vi "ICCD Noise Data Viewer.vi"() -> ()   [LabVIEW 2021, in "AlliGator Camera Noise Influence on Lifetime.lvlib"]
uses:
  AlliGator Camera Noise Influence on Lifetime.lvlib
  Decay Fit Parameter Map/AlliGator Power Law Fit Results.ctl
  Power Law Parameters.ctl
  ICCD Parameter Set.ctl
  Utilities/Utilities.lvlib
  Graphs/XY Graph/XY Graph Add-Ons.lvlib
  <vilib>/Utility/miscctls.llb/LVPoint32TypeDef.ctl
  Graphs/XY Graph/XY Graph Event.ctl
panel:
  out "LabVIEW PL+B":T1={"Power Law Parameters"={"amplitude"=1354.9125948149328, "power"=-1.4827495284911292, "offset"=0.013950226554821962}, "R^2"=0.9896721333021318, "Chi^2"=0.00026681950170242603}
  in  "Abscissa":enum32{"I-", "<I>"}(radio)=enum."<I>"
  out "error out":T3
  out "Data":T1={"Power Law Parameters"={"amplitude"=20.050788088429826, "power"=-0.808279791250982, "offset"=0.0}, "R^2"=0.9320325995197519, "Chi^2"=0.0015050842644887775}
  out "LabVIEW PL":T1={"Power Law Parameters"={"amplitude"=1354.9125919047456, "power"=-1.4228141762361315, "offset"=0.0}, "R^2"=0.6411917195333446, "Chi^2"=0.007945525253030357}
  out "File Name":string="Bin1_MCP560_Power300_Exp100_alligator_sliced"
  out "XY Graph":cluster{"X Array":dbl[], "Y Array":dbl[]}[](graph)=[{"X Array"=[589.8712230215828, 1449.84, 2492.5444234404536, 3505.6867469879517, 4503.983673469388, 5488.8125, 6478.855626326964, 7416.982608695652, 8415.288], "Y Array"=[0.12017889524722658, 0.04584267100112674, 0.02646477188778284, 0.021275407414964982, 0.018663783988422344, 0.018541333295241307, 0.013827404460717034, 0.016008850611953694, 0.01898370316876584]}, {"X Array"=[589.8712230215828, 1449.84, 2492.5444234404536, 3505.6867469879517, 4503.983673469388, 5488.8125, 6478.855626326964, 7416.982608695652, 8415.288], "Y Array"=[0.1155004849822888, 0.05583411708587998, 0.03603237727021303, 0.027350309068035653, 0.022335836275987765, 0.019036444971124028, 0.01664844199637044, 0.01492464998854605, 0.013476486701475781]}, {"X Array"=[589.8712230215828, 1449.84, 2492.5444234404536, 3505.6867469879517, 4503.983673469388, 5488.8125, 6478.855626326964, 7416.982608695652, 8415.288], "Y Array"=[0.15475284512882467, 0.04304673899987971, 0.019912216190079178, 0.012256256772752168, 0.008580684756946514, 0.0064763215930010035, 0.005115139257444052, 0.0042198505196813525, 0.0035258796664633094]}, {"X Array"=[589.8712230215828, 1449.84, 2492.5444234404536, 3505.6867469879517, 4503.983673469388, 5488.8125, 6478.855626326964, 7416.982608695652, 8415.288], "Y Array"=[0.11952795988993804, 0.041777164889661475, 0.026410874061133384, 0.021464735869369332, 0.019132762657076766, 0.017815688947243814, 0.016973058263863076, 0.01642385025852421, 0.016001469474992334]}]
  in  "MCP Voltage (V)":i32(ring)=2 items=["460", "510", "560", "610"]
  in  "Laser Power (mW)":i32(ring)=2 items=["100", "200", "300", "400", "500", "600"]
  in  "Exposure (ms)":i32(ring) items=["100", "200", "300", "400", "500"]
  in  "Binning":i32(ring) items=["1", "2", "4"]
  in  "Analysis Data Folder":path=path "D:/UCLA Thinkpad Google Drive/Work/Manuscripts/2025/OL 2025 (ICCD Lifetime CV)/Material/Intensity sliced"
  in  "Parameter File":path=path "D:/UCLA Thinkpad Google Drive/Work/Manuscripts/2025/OL 2025 (ICCD Lifetime CV)/Material/LUT.xlsx"
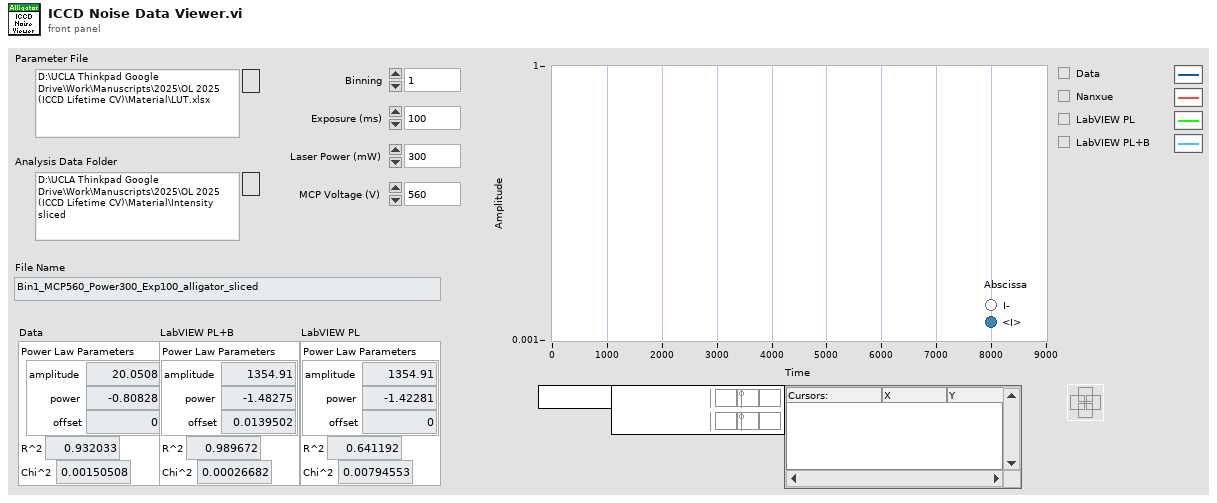
[diagram p1: front panel]
types:
  T1 = typedef "AlliGator Camera Noise Influence on Lifetime.lvlib/AlliGator Power Law Fit Results.ctl" = cluster{"Power Law Parameters":T2, "R^2":dbl, "Chi^2":dbl}
  T2 = typedef "AlliGator Camera Noise Influence on Lifetime.lvlib/Power Law Parameters.ctl" = cluster{"amplitude":dbl, "power":dbl, "offset":dbl}
  T3 = cluster{"status":bool, "Error Code":i32, "source":string}
  T4 = typedef "XY Graph Add-Ons.lvlib/XY Graph Event.ctl" = cluster{"Item Tag":string, "XY Graph Refnum":refnum<vi>, "Coords":T5, "Item Path":string}
  T5 = typedef "LVPoint32TypeDef.ctl" = cluster{"Horizontal":i32, "Vertical":i32}
  T6 = typedef "AlliGator Camera Noise Influence on Lifetime.lvlib/ICCD Parameter Set.ctl" = cluster{"Binning":refnum<vi>, "Exposure (ms)":refnum<vi>, "Laser Power (mW)":refnum<vi>, "MCP Voltage (V)":refnum<vi>}
  T7 = typedef "XY Graph Add-Ons.lvlib/XY Graph Plot Data.ctl" = cluster{"X Array":dbl[], "Y Array":dbl[]}
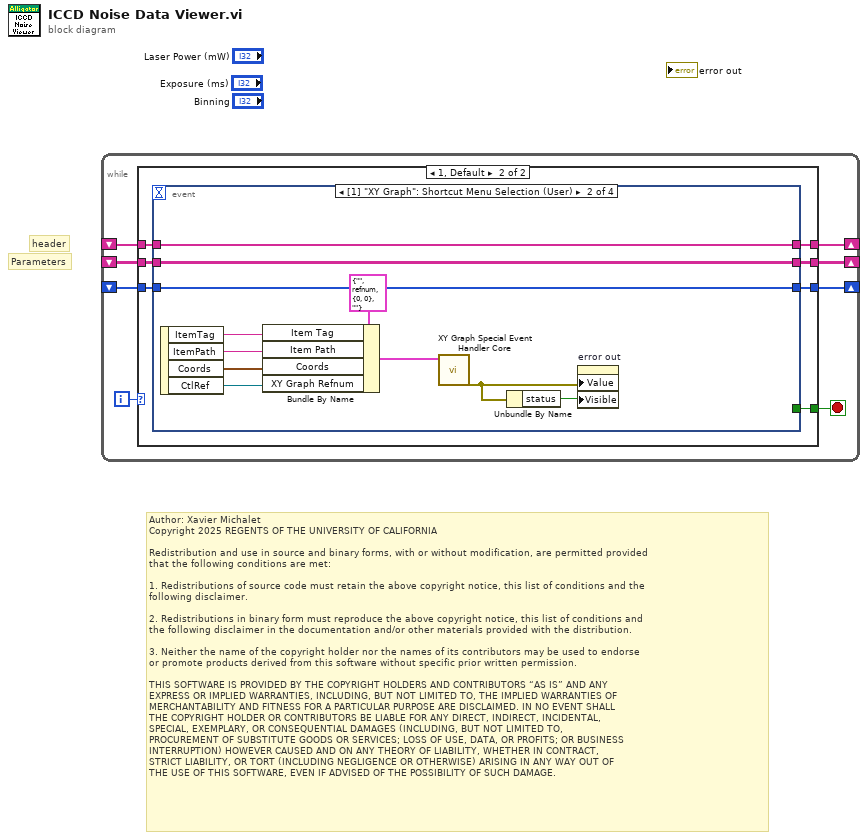
[diagram p0: block diagram]
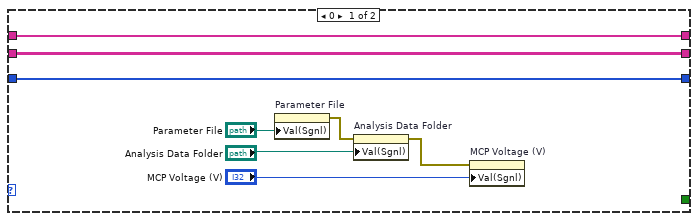
[diagram p2: hidden frame]
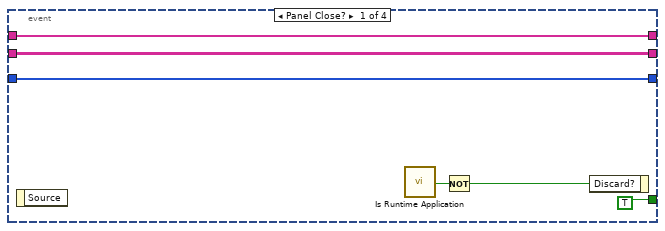
[diagram p3: hidden frame]
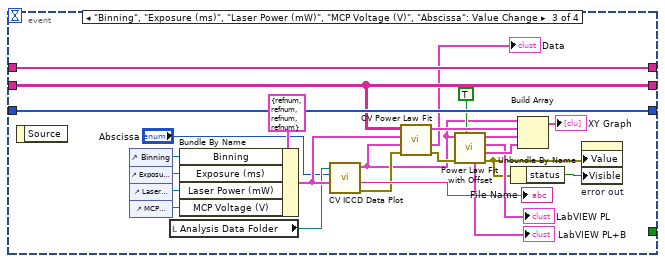
[diagram p4: hidden frame]
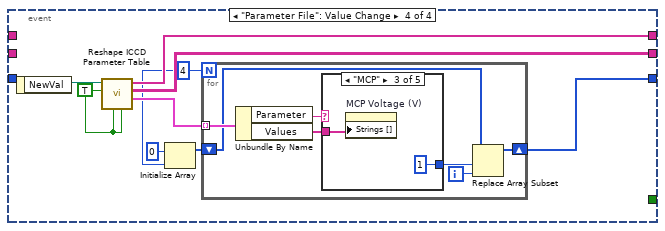
[diagram p5: hidden frame]
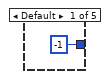
[diagram p6: hidden frame]
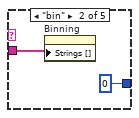
[diagram p7: hidden frame]
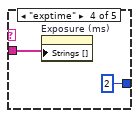
[diagram p8: hidden frame]
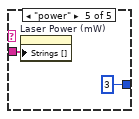
[diagram p9: hidden frame]
diagram:
  # "Author: Xavier Michalet\nCopyright 2025 REGENTS OF THE UNIVERSITY OF CALIFORNIA\n\nRedistribution and use in source and binary forms, with or without modification, are permitted provided\nthat the following conditions are met:\n\n1. Redistributions of source code must retain the above copyright notice, this list of conditions and the\nfollowing disclaimer.\n\n2. Redistributions in binary form must reproduce the above copyright notice, this list of conditions and\nthe following disclaimer in the documentation and/or other materials provided with the distribution.\n\n3. Neither the name of the copyright holder nor the names of its contributors may be used to endorse \nor promote products derived from this software without specific prior written permission.\n\nTHIS SOFTWARE IS PROVIDED BY THE COPYRIGHT HOLDERS AND CONTRIBUTORS “AS IS” AND ANY \nEXPRESS OR IMPLIED WARRANTIES, INCLUDING, BUT NOT LIMITED TO, THE IMPLIED WARRANTIES OF\nMERCHANTABILITY AND FITNESS FOR A PARTICULAR PURPOSE ARE DISCLAIMED. IN NO EVENT SHALL\nTHE COPYRIGHT HOLDER OR CONTRIBUTORS BE LIABLE FOR ANY DIRECT, INDIRECT, INCIDENTAL, \nSPECIAL, EXEMPLARY, OR CONSEQUENTIAL DAMAGES (INCLUDING, BUT NOT LIMITED TO, \nPROCUREMENT OF SUBSTITUTE GOODS OR SERVICES; LOSS OF USE, DATA, OR PROFITS; OR BUSINESS\nINTERRUPTION) HOWEVER CAUSED AND ON ANY THEORY OF LIABILITY, WHETHER IN CONTRACT, \nSTRICT LIABILITY, OR TORT (INCLUDING NEGLIGENCE OR OTHERWISE) ARISING IN ANY WAY OUT OF\nTHE USE OF THIS SOFTWARE, EVEN IF ADVISED OF THE POSSIBILITY OF SUCH DAMAGE."
  # "Parameters"
  # "header"
  n1 = while {
    shift-right: [w7] -> _
    shift-left: _ -> [w3]
    shift-right: [w6] -> _
    shift-left: _ -> [w4]
    shift-right: [w5] -> _
    shift-left: _ -> [w2]
    i -> [w1]
    stop <- w8 stop-if-true
    n2 = case shown="1, Default" w1 {
      tunnel: [_ w23] -> w8
      tunnel: [w10 w22] -> w7
      tunnel: [w11 w21] -> w6
      tunnel: [w9 w20] -> w5
      tunnel: w4 -> [w11 w19]
      tunnel: w3 -> [w10 w18]
      tunnel: w2 -> [w9 w17]
      frame 0 {
        n3 = property on="Parameter File" class="Path"("Val(Sgnl)"="Parameter File") -> (error out=w15:errorcluster)  [unwired: 2 in, 1 out]
        n4 = property on="Analysis Data Folder" class="Path"(error in=w15, "Val(Sgnl)"="Analysis Data Folder") -> (error out=w16:errorcluster)  [unwired: 1 in, 1 out]
        n5 = property on="MCP Voltage (V)" class="Ring (strict)"(error in=w16, "Val(Sgnl)"="MCP Voltage (V)") -> ()  [unwired: 1 in, 2 out]
      }
      frame 1, Default {
        n6 = event shown="[1] \"XY Graph\": Shortcut Menu Selection (User)" {
          selector: _ -> [_ _ _ _]
          dyn-events: _ -> [_ _ _ _]
          timeout: _ -> [_ _ _ _]
          tunnel: [TRUE ("Discard?") _ _ _] -> w23
          tunnel: [w27 w40 w56 w73] -> w22
          tunnel: [w28 w39 w61 w72] -> w21
          tunnel: [w26 w38 w62 w67] -> w20
          tunnel: w19 -> [w28 w39 w61 _]
          tunnel: w18 -> [w27 w40 w56 _]
          tunnel: w17 -> [w26 w38 w62 _]
          event Panel Close? {
            n7 = event-data() -> ()  [unwired: 1 in, 1 out]
            n8 = call "Is Runtime Application.vi"() -> ("Runtime ?"=w25:bool)  [unwired: 8 in, 1 out]
            n9 = Not(x=w25) -> (.not. x?=w24:bool)
            n10 = event-data("Discard?"=w24) -> ()  [unwired: 1 in, 1 out]
          }
          event "XY Graph": Shortcut Menu Selection (User) {
            n11 = event-data() -> ("ItemTag"=w36:string, "ItemPath"=w35:string, "Coords"=w34:T5, "CtlRef"=w33:refnum<vi>)  [unwired: 1 in]
            n12 = Bundle By Name(cluster=T4 {"Item Tag"="", "XY Graph Refnum"=refnum, "Coords"={"Horizontal"=0, "Vertical"=0}, "Item Path"=""} ("XY Graph Event"), "Item Tag"=w36, "Item Path"=w35, "Coords"=w34, "XY Graph Refnum"=w33) -> (w32:T4)
            n13 = call "XY Graph Special Event Handler Core.vi"("XY Graph Event"=w32) -> ("error out"=w31:errorcluster)  [unwired: 6 in, 4 out]
            n14 = Unbundle By Name(w31) -> ("status"=w30:bool)
            n15 = property on="error out" class="Clust (strict)"("Value"=w31, "Visible"=w30) -> ()  [unwired: 2 in, 2 out]
          }
          event "Binning", "Exposure (ms)", "Laser Power (mW)", "MCP Voltage (V)", "Abscissa": Value Change {
            n16 = event-data() -> ()  [unwired: 1 in, 1 out]
            n17 = control-ref of="Binning"() -> (w60:refnum<vi>)
            n18 = control-ref of="Exposure (ms)"() -> (w59:refnum<vi>)
            n19 = control-ref of="Laser Power (mW)"() -> (w58:refnum<vi>)
            n20 = control-ref of="MCP Voltage (V)"() -> (w57:refnum<vi>)
            n21 = local read "Analysis Data Folder"() -> (w54:path)
            n22 = Bundle By Name(cluster=T6 {"Binning"=refnum, "Exposure (ms)"=refnum, "Laser Power (mW)"=refnum, "MCP Voltage (V)"=refnum} ("output cluster"), "Binning"=w60, "Exposure (ms)"=w59, "Laser Power (mW)"=w58, "MCP Voltage (V)"=w57) -> (w55:T6)
            n23 = call "CV ICCD Data Plot.vi"("ICCD Parameter Set"=w55, "Abscissa"="Abscissa", "Analysis Data Folder"=w54) -> ("Error Out"=w52:errorcluster, "File Name"=→"File Name":string, "Plot"=w43:T7)  [unwired: 5 in, 1 out]
            n24 = call "CV Power Law Fit.vi"("Error In"=w52, "Plot"=w43, "ICCD Parameter Set"=w55, "ICCD Parameter Array"=w56) -> ("Error Out"=w50:errorcluster, "Power Law Fit Results"=→"Data":T1, "Plot Fit"=w63:T7)  [unwired: 5 in]
            n25 = call "Power Law Fit with Offset.vi"("Poisson Weight"=TRUE, "Error In"=w50, "Plot"=w43) -> ("Error Out"=w42:errorcluster, "Power Law with Baseline Fit"=w47:T7, "Power Law Fit Results"=→"LabVIEW PL":T1, "Power Law Fit"=w51:T7, "Power Law + Baselien Fit Results"=→"LabVIEW PL+B":T1)  [unwired: 4 in]
            n26 = Unbundle By Name(w42) -> ("status"=w41:bool)
            n27 = Build Array(w43, w63, w51, w47) -> (→"XY Graph":T7[])
            n28 = property on="error out" class="Clust (strict)"("Value"=w42, "Visible"=w41) -> ()  [unwired: 2 in, 2 out]
          }
          event "Parameter File": Value Change {
            w66 = TRUE ("Repeat multicell values (F)?")
            w69 = 4
            n29 = event-data() -> ("NewVal"=w74:path)  [unwired: 1 in]
            n30 = call "Reshape ICCD Parameter Table.vi"("Remove empty rows (F)?"=w66, "Remove empty columns (F)?"=w66, "Repeat multicell values (F)?"=w66, "XLSX File"=w74) -> ("Parameter Values"=w71:cluster{"Parameter":string, "Values":string[]}[], "ICCD Parameter Array"=w73:string[][], "Header"=w72:string[])  [unwired: 4 in, 1 out]
            n31 = Initialize Array(0, w69) -> (w68:i32[])
            n32 = for {
              N: w69 -> [_]
              tunnel: w71 -> [w80] mode=indexing
              shift-right: [w75] -> w67
              shift-left: w68 -> [w78]
              i -> [w77]
              n33 = Unbundle By Name(w80) -> ("Parameter"=w79:string, "Values"=w81:string[])
              n34 = case shown="\"MCP\"" w79 {
                tunnel: w81 -> [_ w84 w86 w88 w90]
                tunnel: [-1 ("index") 0 ("index") 1 ("index") 2 ("index") 3 ("index")] -> w76
                frame Default {
                }
                frame "bin" {
                  n35 = property on="Binning" class="Ring (strict)"("Strings []"=w84) -> ()  [unwired: 2 in, 2 out]
                }
                frame "MCP" {
                  n36 = property on="MCP Voltage (V)" class="Ring (strict)"("Strings []"=w86) -> ()  [unwired: 2 in, 2 out]
                }
                frame "exptime" {
                  n37 = property on="Exposure (ms)" class="Ring (strict)"("Strings []"=w88) -> ()  [unwired: 2 in, 2 out]
                }
                frame "power" {
                  n38 = property on="Laser Power (mW)" class="Ring (strict)"("Strings []"=w90) -> ()  [unwired: 2 in, 2 out]
                }
              }
              n39 = Replace Array Subset(array=w78, new element=w77, index=w76) -> (w75:i32[])
            }
          }
        }
      }
    }
  }
